vi "Gaussian Peak Fit (Bisquare).vi"(0 "Y":dbl[](array[numeric]), 5 "X":dbl[](array[numeric]), 7 "Weight":dbl[](array[numeric]), 9 "tolerance":dbl=-1.0 format="%#_3g", 11 "Initial Coefficients":dbl[](array[numeric])) -> (4 "Best Gaussian Fit":dbl[](array[numeric]), 6 "amplitude":dbl, 8 "center":dbl, 10 "width":dbl, 14 "residue":dbl, 15 "error":i32)   [LabVIEW 2017, in "NI_AALPro.lvlib"]
uses:
  NI_AALPro.lvlib
  <resource>/lvanlys.dll
panel:
  # "Bisquare Gaussian Peak Fit"
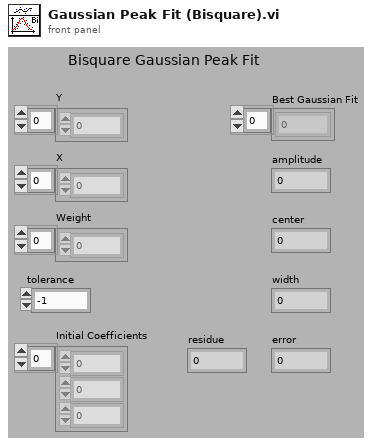
[diagram p1: front panel]
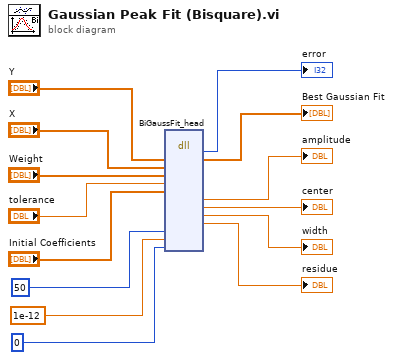
[diagram p0: block diagram]
diagram:
  n1 = dll-call lib="C:/Program Files (x86)/National Instruments/LabVIEW 2017/resource/lvanlys.*" fn="BiGaussFit_head"("y"="Y", "x"="X", "weight"="Weight", "tolerance"="tolerance", "initialCoef"="Initial Coefficients", "maxIter"=50, "absTol"=1e-12, "isCoef"=0) -> (→"error":i32, "y"=→"Best Gaussian Fit":dbl[], "amp"=→"amplitude":dbl, "center"=→"center":dbl, "width"=→"width":dbl, "meanErr"=→"residue":dbl)  [unwired: 14 in, 2 out]
